vi "TestCase_ShellInit.vi"(8 "error in (no error)":errorcluster, 10 "methodPath (\"testXXX\")":path, 11 "TestCase in":refnum<class "TestCase.lvclass">) -> (0 "error out":errorcluster, 3 "TestCase out":refnum<class "TestCase.lvclass">)   [LabVIEW 2013, in "TestCase.lvclass"]
uses:
  TestCase.lvclass
  TestCase.lvclass/TestCase.ctl
  <userlib>/_OpenG.lib/file/file.llb/Strip Path Extension - String__ogtk.vi
panel:
  # "JKI VI Tester for LabVIEW\nhttp://jkisoft.com/vi-tester\nCopyright (C) 2007-2009, JKI <info@jkisoft.com>\nALL RIGHTS RESERVED"
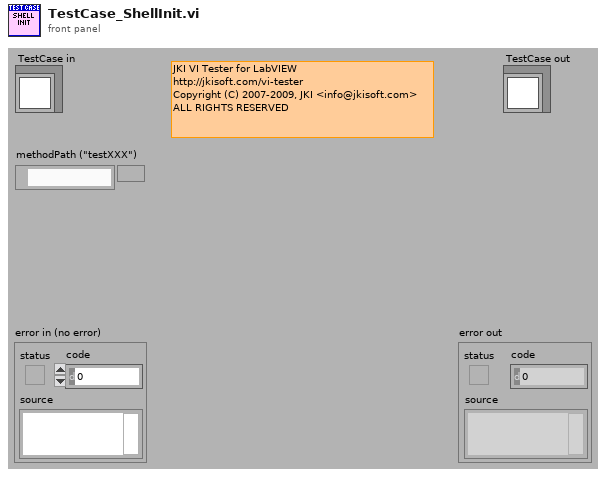
[diagram p1: front panel]
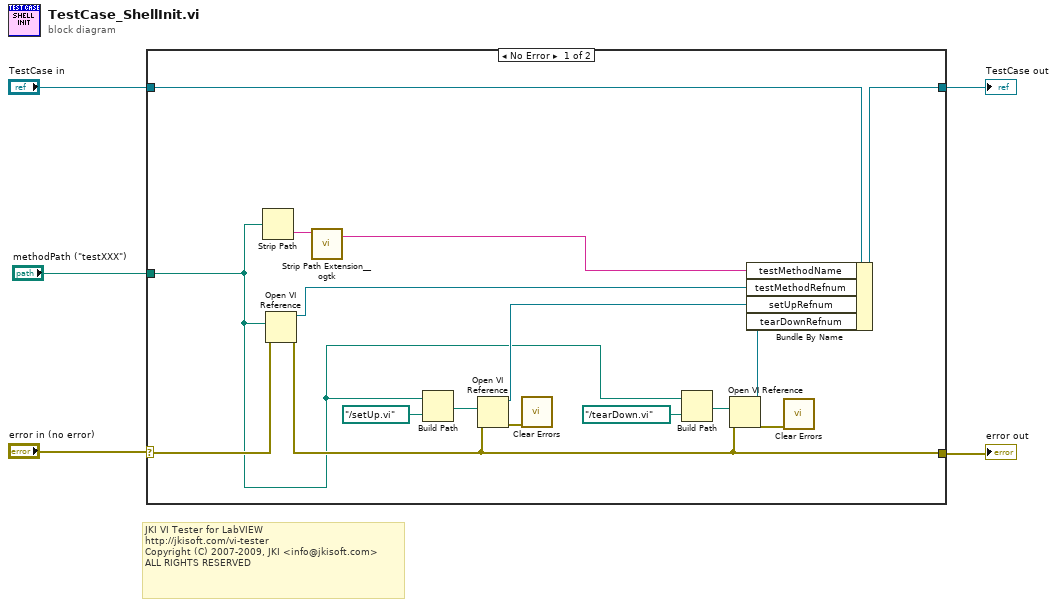
[diagram p0: block diagram]
diagram:
  # "JKI VI Tester for LabVIEW\nhttp://jkisoft.com/vi-tester\nCopyright (C) 2007-2009, JKI <info@jkisoft.com>\nALL RIGHTS RESERVED"
  n1 = case shown="No Error" "error in (no error)" {
    selector: "error in (no error)" -> [w18 w22]
    tunnel: "TestCase in" -> [w19 w23]
    tunnel: [w21 w23] -> w4
    tunnel: [w9 w22] -> w2
    tunnel: "methodPath (\"testXXX\")" -> [w6 _]
    frame No Error {
      n2 = Strip Path(path=w6) -> (name=w17:string)  [unwired: 1 out]
      n3 = Open VI Reference(vi path=w6, error in (no error)=w18) -> (vi reference=w20:refnum<vi>, error out=w9:errorcluster)  [unwired: 4 in]
      n4 = call-poly <userlib>:"Strip Path Extension__ogtk.vi"("path"=w17) -> ("root"=w16:string)  [unwired: 1 out]
      n5 = Build Path(base path=w6, name or relative path=path "../setUp.vi") -> (appended path=w14:path)
      n6 = Open VI Reference(vi path=w14, error in (no error)=w9) -> (vi reference=w8:refnum<vi>, error out=w10:errorcluster)  [unwired: 4 in]
      n7 = call <vilib>:"Clear Errors.vi"("error in (no error)"=w10) -> ()  [unwired: 6 in, 1 out]
      n8 = Build Path(base path=w6, name or relative path=path "../tearDown.vi") -> (appended path=w13:path)
      n9 = Open VI Reference(vi path=w13, error in (no error)=w9) -> (vi reference=w7:refnum<vi>, error out=w11:errorcluster)  [unwired: 4 in]
      n10 = Bundle By Name(cluster=w19, "testMethodName"=w16, "testMethodRefnum"=w20, "setUpRefnum"=w8, "tearDownRefnum"=w7) -> (w21:refnum<class "TestCase.lvclass">)
      n11 = call <vilib>:"Clear Errors.vi"("error in (no error)"=w11) -> ()  [unwired: 6 in, 1 out]
    }
    frame Error {
    }
  }
  "TestCase out" <- w4
  "error out" <- w2
